vi "Get All Logger Info.vi"(8 "error in":errorcluster) -> (0 "error out":errorcluster, 3 "logger info":T2(array[cluster]))   [LabVIEW 2018, in "GLog.lvlib" / "Registry.lvlib"]
uses:
  Registry.lvlib
  api/Log Levels.ctl
  Registry Actions.ctl
  reuse_library/Utilities/Utilities.lvlib
  api/GLog.lvlib
panel:
  # "Connector Pane"
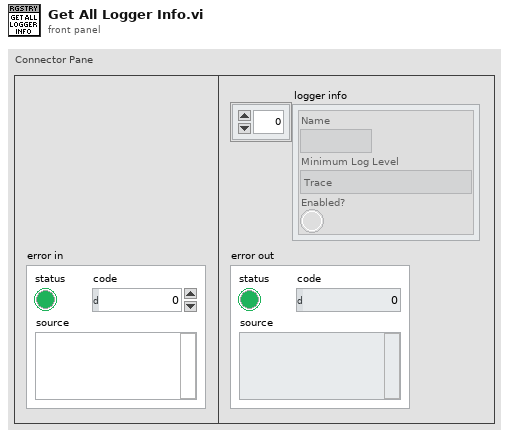
[diagram p1: front panel]
types:
  T1 = typedef "GLog.lvlib/Log Levels.ctl" = enum16{"Trace", "Debug", "Info", "Warning", "Error", "Critical"}
  T2 = cluster{"Name":string, "Minimum Log Level":T1, "Enabled?":bool}[]
  T3 = cluster{"name":string, "minimum log level":T1, "Enabled?":bool}[]
  T4 = typedef "GLog.lvlib/Registry.lvlib/Registry Actions.ctl" = enum16{"Register", "Log", "Enable", "Enable All", "Disable", "Disable All", "Get Enable State", "Get Minimum Log Level", "Set Minimum Log Level", "Set All Minimum Log Level", "Get Logger Info", "Get All Logger Info", "List", "Unregister", "Unregister All", "Shutdown"}
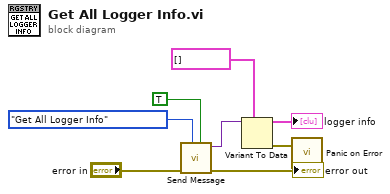
[diagram p0: block diagram]
diagram:
  n1 = call "Send Message.vi"("return data? (F)"=TRUE, "action"=Registry_Actions."Get All Logger Info", "error in (no error)"="error in") -> ("error out"=→"error out":errorcluster, "return data"=w3:variant)  [unwired: 7 in]
  n2 = Variant To Data(type=T3 [], Variant=w3) -> (data=→"logger info":T3, error out=w4:errorcluster)  [unwired: 1 in]
  n3 = call "Panic on Error.vi"("error in (no error)"=w4) -> ()  [unwired: 3 in]
